vi "温度显示数值控件.vi"() -> ()   [LabVIEW 2012]
panel:
  in  "选择":bool
  out "测量温度":dbl format="%.2f ℉"
  out "格式字符串":string
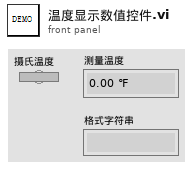
[diagram p1: front panel]
types:
  T1 = typedef "特殊单位符号菜单列表.ctl" = u16
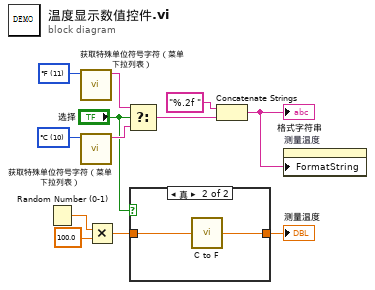
[diagram p0: block diagram]
diagram:
  w8 = T1 11 items=["°", "′", "″", "＄", "￥", "〒", "￠", "￡", "％", "＠", "℃", "℉", "﹩", "﹪", "‰", "﹫", "㏕", "㎜", "㎝", "㎞", "㏎", "㎡", "㎎", "㎏", "㏄", "°", "○", "¤", ""] ("特殊单位符号")
  w12 = T1 10 items=["°", "′", "″", "＄", "￥", "〒", "￠", "￡", "％", "＠", "℃", "℉", "﹩", "﹪", "‰", "﹫", "㏕", "㎜", "㎝", "㎞", "㏎", "㎡", "㎎", "㎏", "㏄", "°", "○", "¤", ""] ("特殊单位符号")
  n1 = Random Number (0-1)() -> (number: 0 to 1=w11:dbl)
  n2 = call "获取特殊单位符号字符（菜单下拉列表）.vi"("特殊单位符号"=w8) -> ("字符（双字节）"=w7:string)  [unwired: 10 in]
  n3 = call "获取特殊单位符号字符（菜单下拉列表）.vi"("特殊单位符号"=w12) -> ("字符（双字节）"=w6:string)  [unwired: 10 in]
  n4 = Multiply(x=w11, y=100.0) -> (x*y=w9:dbl)
  n5 = Select(t=w7, s="选择", f=w6) -> (s? t:f=w4:string)
  n6 = case shown="真" "选择" {
    tunnel: w9 -> [w13 w15]
    tunnel: [w13 w14] -> w2
    frame False {
    }
    frame True {
      n7 = call-poly "C to F.vi"("C"=w15) -> ("F"=w14:dbl)
    }
  }
  "测量温度" <- w2
  n8 = Concatenate Strings("%.2f " ("字符串"), w4) -> (w1:string)
  "格式字符串" <- w1
  n9 = property on="测量温度" class="DigNum (严格)"("FormatString"=w1) -> ()  [unwired: 2 in, 2 out]
